vi "DB- HWIO Config.vi"(6 "Enum":T1(ring)=enum."Read", 8 "error in (no error)":errorcluster, 9 "Database table":string[][](table), 11 "columns Header":string[](array[string])=["SerialNo", "ControlChannel", "FeedbackChannel"]) -> (0 "error out":errorcluster, 2 "Read Databaase":string[][](array[string]), 3 "data":string[][](array[string]))   [LabVIEW 2015]
uses:
  <vilib>/addons/database/Connection.llb/DB Tools Open Connec (String).vi
  <vilib>/addons/database/_DB Variant To Data/Database Variant To Data.xnode
  <vilib>/addons/database/NI_Database_API.lvlib
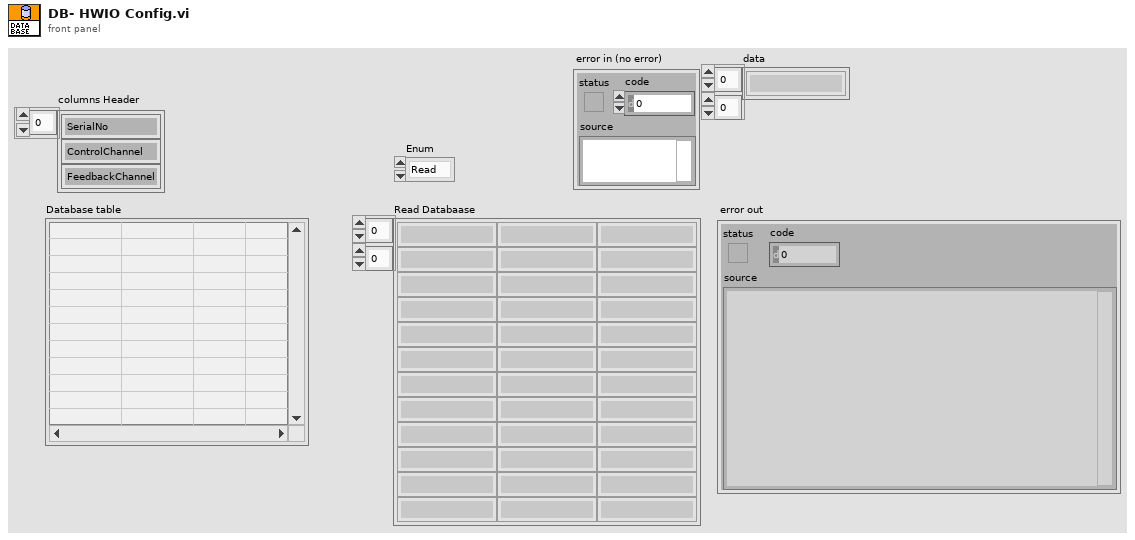
[diagram p1: front panel]
types:
  T1 = enum16{"Selection", "Insert Data", "Edit", "Read"}
  T2 = typedef "NI_Database_API.lvlib/Conn ObjectReference.ctl" = refnum<k1>
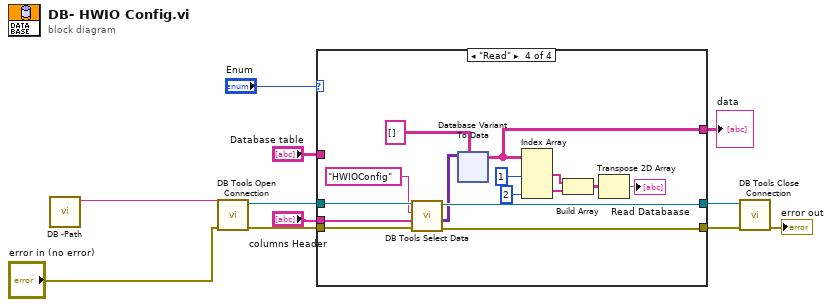
[diagram p0: block diagram]
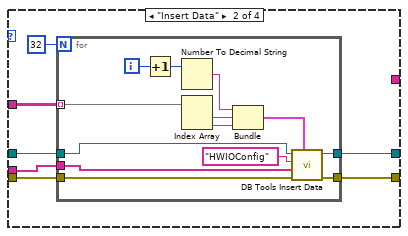
[diagram p3: hidden frame]
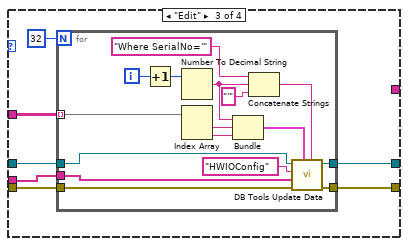
[diagram p4: hidden frame]
diagram:
  n1 = call "DB -Path.vi"() -> ("String"=w1:string)  [unwired: 11 in]
  n2 = call-poly <vilib>:"DB Tools Open Connection.vi"("error in (no error)"="error in (no error)", "connection information"=w1) -> ("error out"=w5:errorcluster, "connection reference"=w6:T2)  [unwired: 6 in]
  n3 = case shown="\"Read\"" "Enum" {
    tunnel: "Database table" -> [_ w20 w38 _]
    tunnel: "columns Header" -> [_ w19 w40 w69]
    tunnel: [w12 w18 w36 w66] -> w8
    tunnel: [w13 w17 w37 w67] -> w7
    tunnel: w6 -> [w13 w16 w35 w71]
    tunnel: w5 -> [w12 w15 w34 w70]
    tunnel: [_ _ _ w57] -> w2
    frame "Selection", Default {
    }
    frame "Insert Data" {
      n4 = for {
        N: 32 -> [_]
        tunnel: w16 -> [w33]
        tunnel: w15 -> [w32]
        tunnel: w20 -> [w28] mode=indexing
        tunnel: [w30] -> w17
        tunnel: [w29] -> w18
        tunnel: w19 -> [w24]
        i -> [w21]
        n5 = Increment(x=w21) -> (x+1=w23:i32)
        n6 = Number To Decimal String(number=w23) -> (decimal integer string=w22:string)  [unwired: 1 in]
        n7 = Index Array(array=w28) -> (element #1=w27:string, element #2=w26:string)  [unwired: 2 in]
        n8 = Bundle(w22, w27, w26) -> (w25:cluster{string, string, string})  [unwired: 1 in]
        n9 = call <vilib>:"DB Tools Insert Data.vi"("data"=w25, "error in (no error)"=w32, "columns"=w24, "table"="HWIOConfig", "connection reference"=w33) -> ("error out"=w29:errorcluster, "connection reference out"=w30:T2)  [unwired: 5 in]
      }
    }
    frame "Edit" {
      n10 = for {
        N: 32 -> [_]
        tunnel: w40 -> [w56]
        tunnel: w38 -> [w47] mode=indexing
        tunnel: [w44] -> w37
        tunnel: [w43] -> w36
        tunnel: w35 -> [w42]
        tunnel: w34 -> [w41]
        i -> [w53]
        n11 = Increment(x=w53) -> (x+1=w52:i32)
        n12 = Number To Decimal String(number=w52) -> (decimal integer string=w46:string)  [unwired: 1 in]
        n13 = Index Array(array=w47) -> (element #1=w49:string, element #2=w48:string)  [unwired: 2 in]
        n14 = Bundle(w46, w49, w48) -> (w45:cluster{string, string, string})  [unwired: 1 in]
        n15 = Concatenate Strings("Where SerialNo='" ("condition"), w46, "'" ("string")) -> (w50:string)
        n16 = call <vilib>:"DB Tools Update Data.vi"("condition"=w50, "data"=w45, "error in (no error)"=w41, "columns"=w56, "table"="HWIOConfig", "connection reference"=w42) -> ("error out"=w43:errorcluster, "connection reference out"=w44:T2)  [unwired: 4 in]
      }
    }
    frame "Read" {
      n17 = call <vilib>:"DB Tools Select Data.vi"("error in (no error)"=w70, "columns"=w69, "table"="HWIOConfig", "connection reference"=w71) -> ("error out"=w66:errorcluster, "data"=w65:variant[][], "connection reference out"=w67:T2)  [unwired: 2 in]
      n18 = xnode "Database Variant To Data"("database variant"=w65, "type"=string[][] []) -> ("data"=w57:string[][])  [unwired: 1 in, 1 out]
      n19 = Index Array(array=w57, index (col) #1=1 ("disabled index (col)"), index (col) #2=2 ("disabled index (col)")) -> (element #1=w61:string[], element #2=w60:string[])  [unwired: 2 in]
      n20 = Build Array(w61, w60) -> (w59:string[][])
      n21 = Transpose 2D Array(2D array=w59) -> (transposed array=→"Read Databaase":string[][])
    }
  }
  "data" <- w2
  n22 = call <vilib>:"DB Tools Close Connection.vi"("error in (no error)"=w8, "connection reference"=w7) -> ("error out"=→"error out":errorcluster)  [unwired: 5 in]
